vi "Init Msg Default.vi"() -> (3 "TEMPLATE Msg out":refnum<class "TEMPLATE Msg.lvclass">)   [LabVIEW 2025, in "_Template.lvlib" / "Templates.lvlib" / "TEMPLATE jettl Msg.lvlib" / "TEMPLATE Msg.lvlib" / "TEMPLATE Msg.lvclass"]
uses:
  TEMPLATE Msg.lvclass
  TEMPLATE Msg.lvclass/TEMPLATE Msg.ctl
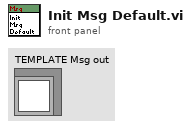
[diagram p1: front panel]
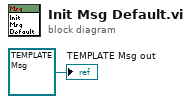
[diagram p0: block diagram]
diagram:
  "TEMPLATE Msg out" <- refnum<class "TEMPLATE Msg.lvclass"> refnum ("TEMPLATE Msg out")
